vi "Microphone Board Test.vi"(7 "Test Configuration":T2, 8 "error in (no error)":errorcluster, 11 "Session Handle in":T1) -> (0 "error out":errorcluster, 1 "Failure Reason":string, 2 "Success?":bool, 3 "Session Handle out":T1 caption="Gas")   [LabVIEW 2015, in "PAS.lvclass"]
uses:
  PAS.lvclass
  Typedefs/Session Handle.ctl
  Tests/Controls/Test Configuration.ctl
  Tests/Controls/Vacuum Test.ctl
  Tests/Controls/Test Timing.ctl
  Tests/Controls/Vaccum Thresholds.ctl
  Tests/Controls/Helium Test.ctl
  Tests/Controls/Helium Thresholds.ctl
  Tests/Controls/Functional Test.ctl
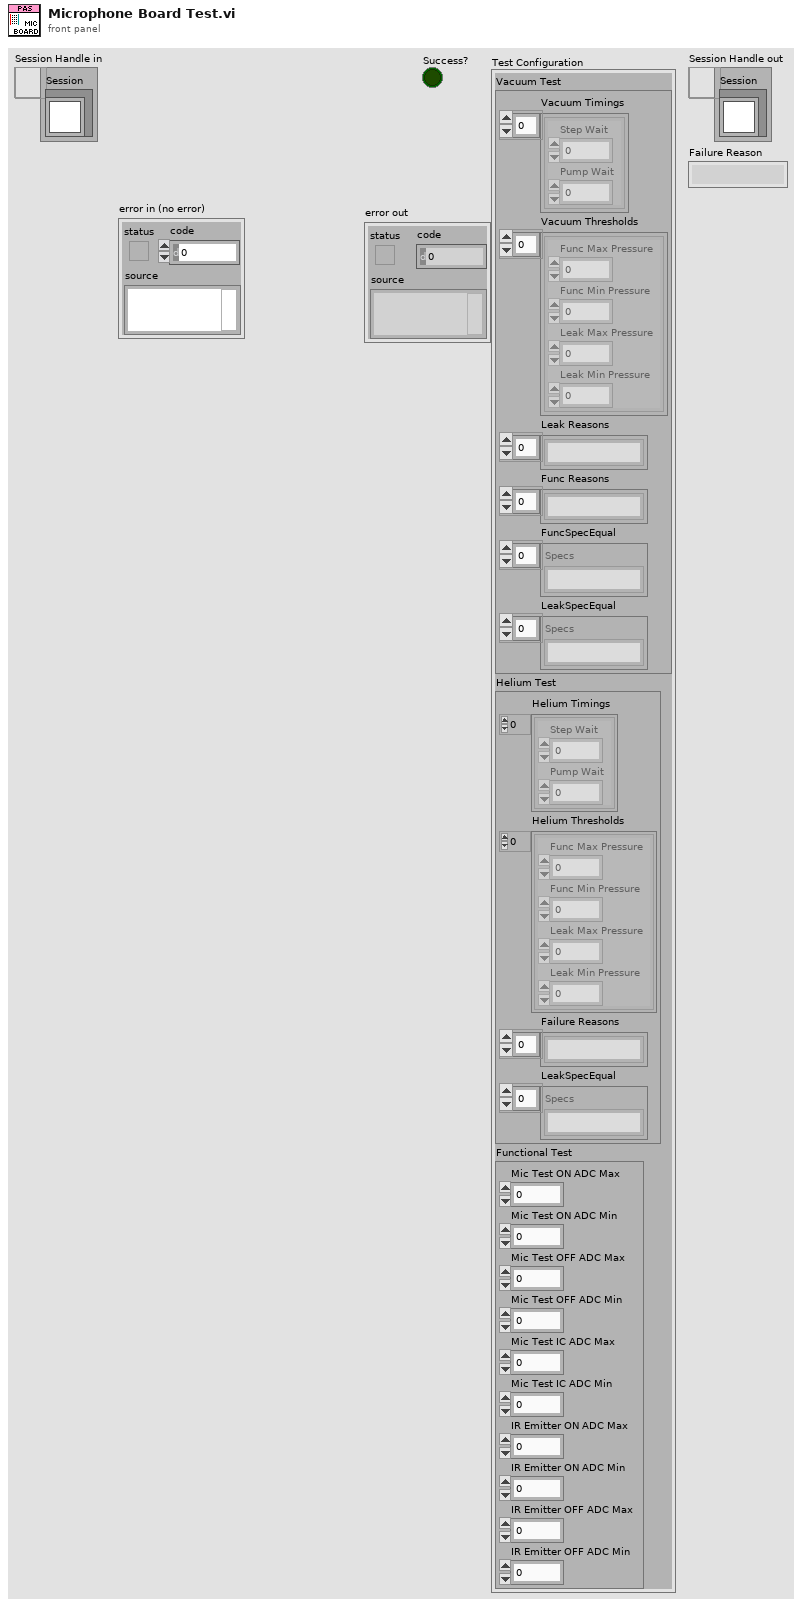
[diagram p1: front panel]
types:
  T1 = typedef "PAS.lvclass/Session Handle.ctl" = refnum<data-value>
  T2 = typedef "Test Configuration.ctl" = cluster{"Vacuum Test":T3, "Helium Test":T6, "Functional Test":T8}
  T3 = typedef "Vacuum Test.ctl" = cluster{"Vacuum Timings":T4[], "Vacuum Thresholds":T5[], "Leak Reasons":string[], "Func Reasons":string[], "FuncSpecEqual":string[], "LeakSpecEqual":string[]}
  T4 = typedef "Test Timing.ctl" = cluster{"Step Wait":dbl, "Pump Wait":dbl}
  T5 = typedef "Vaccum Thresholds.ctl" = cluster{"Func Max Pressure":dbl, "Func Min Pressure":dbl, "Leak Max Pressure":dbl, "Leak Min Pressure":dbl}
  T6 = typedef "Helium Test.ctl" = cluster{"Helium Timings":T4[], "Helium Thresholds":T7[], "Failure Reasons":string[], "LeakSpecEqual":string[]}
  T7 = typedef "Helium Thresholds.ctl" = cluster{"Func Max Pressure":dbl, "Func Min Pressure":dbl, "Leak Max Pressure":dbl, "Leak Min Pressure":dbl}
  T8 = typedef "Functional Test.ctl" = cluster{"Mic Test ON ADC Max":dbl, "Mic Test ON ADC Min":dbl, "Mic Test OFF ADC Max":dbl, "Mic Test OFF ADC Min":dbl, "Mic Test IC ADC Max":dbl, "Mic Test IC ADC Min":dbl, "IR Emitter ON ADC Max":dbl, "IR Emitter ON ADC Min":dbl, "IR Emitter OFF ADC Max":dbl, "IR Emitter OFF ADC Min":dbl}
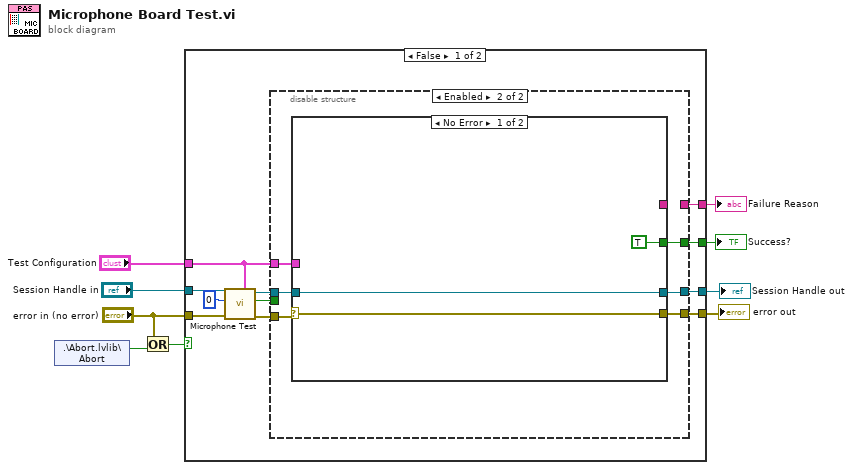
[diagram p0: block diagram]
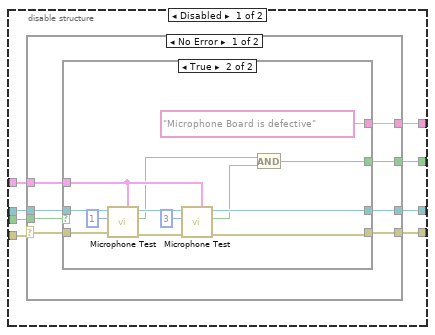
[diagram p2: hidden frame]
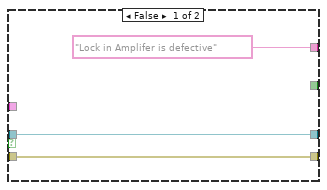
[diagram p3: hidden frame]
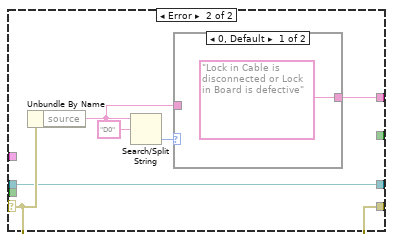
[diagram p4: hidden frame]
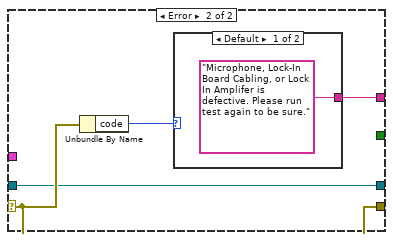
[diagram p6: hidden frame]
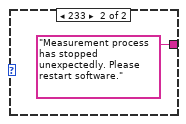
[diagram p7: hidden frame]
diagram:
  n1 = shared-variable ".\\Abort.lvlib\\Abort"() -> (w8:bool)  [unwired: 1 in, 1 out]
  n2 = Or(x="error in (no error)", y=w8) -> (x .or. y?=w9:bool)
  n3 = case shown="False" w9 {
    tunnel: "error in (no error)" -> [w20 w77]
    tunnel: "Session Handle in" -> [w19 w76]
    tunnel: "Test Configuration" -> [w13 _]
    tunnel: [w15 w77] -> w2
    tunnel: [w12 _] -> w4
    tunnel: [w11 w76] -> w3
    tunnel: [w10 _] -> w1
    frame False {
      n4 = call "Microphone Test.vi"("Test Configuration"=w13, "error in (no error)"=w20, "Mic Command"=u8 0, "Session Handle in"=w19) -> ("error out"=w17:errorcluster, "Success?"=w16:bool, "Session Handle out"=w14:T1)  [unwired: 4 in, 1 out]
      n5 = disable-structure shown="Enabled" {
        disable-tunnel: w17 -> [w28 w65]
        disable-tunnel: w16 -> [w27 _]
        disable-tunnel: [w26 w61] -> w15
        disable-tunnel: w14 -> [w25 w64]
        disable-tunnel: w13 -> [w24 w66]
        disable-tunnel: [w23 w62] -> w12
        disable-tunnel: [w22 w63] -> w11
        disable-tunnel: [w21 _] -> w10
        frame Disabled {
          n6 = case shown="No Error" w28 {
            selector: w28 -> [w36 w54]
            tunnel: [w33 w55] -> w21
            tunnel: w27 -> [w35 _]
            tunnel: [w34 w54] -> w26
            tunnel: w25 -> [w32 w53]
            tunnel: w24 -> [w31 _]
            tunnel: [w30 _] -> w23
            tunnel: [w29 w53] -> w22
            frame No Error {
              n7 = case shown="True" w35 {
                tunnel: w36 -> [w39 w52]
                tunnel: [w39 w44] -> w34
                tunnel: ["Lock in Amplifer is defective" ("source") "Microphone Board is defective" ("source")] -> w33
                tunnel: w32 -> [w37 w51]
                tunnel: w31 -> [_ w47]
                tunnel: [w37 w45] -> w29
                tunnel: [_ w41] -> w30
                frame False {
                }
                frame True {
                  n8 = call "Microphone Test.vi"("Test Configuration"=w47, "error in (no error)"=w52, "Mic Command"=u8 1, "Session Handle in"=w51) -> ("error out"=w49:errorcluster, "Success?"=w43:bool, "Session Handle out"=w48:T1)  [unwired: 4 in, 1 out]
                  n9 = call "Microphone Test.vi"("Test Configuration"=w47, "error in (no error)"=w49, "Mic Command"=u8 3, "Session Handle in"=w48) -> ("error out"=w44:errorcluster, "Success?"=w42:bool, "Session Handle out"=w45:T1)  [unwired: 4 in, 1 out]
                  n10 = And(x=w43, y=w42) -> (x .and. y?=w41:bool)
                }
              }
            }
            frame Error {
              n11 = Unbundle By Name(w54) -> ("source"=w56:string)
              n12 = Search/Split String(string=w56, search string/char (-)="D0") -> (offset of match=w57:i32)  [unwired: 1 in, 2 out]
              n13 = case shown="0, Default" w57 {
                tunnel: ["Lock in Cable is disconnected or Lock in Board is defective" ("source") w60] -> w55
                tunnel: w56 -> [_ w60]
                frame 0, Default {
                }
                frame -1 {
                }
              }
            }
          }
        }
        frame Enabled {
          n14 = case shown="No Error" w65 {
            selector: w65 -> [w69 w72]
            tunnel: [_ w73] -> _
            tunnel: [w69 w72] -> w61
            tunnel: w66 -> [_ _]
            tunnel: w64 -> [w68 w71]
            tunnel: [w68 w71] -> w63
            tunnel: [TRUE _] -> w62
            frame No Error {
            }
            frame Error {
              n15 = Unbundle By Name(w72) -> ("code"=w70:i32)
              n16 = case shown="Default" w70 {
                tunnel: ["Microphone, Lock-In Board Cabling, or Lock In Amplifer is defective. Please run test again to be sure." ("source") "Measurement process has stopped unexpectedly. Please restart software." ("source")] -> w73
                frame Default {
                }
                frame 233 {
                }
              }
            }
          }
        }
      }
    }
    frame True {
    }
  }
  "error out" <- w2
  "Success?" <- w4
  "Session Handle out" <- w3
  "Failure Reason" <- w1
